vi "decoupled_gains_vec.vi"(11 "Gain":T1 {"Rz" min=0 max=1 step=0.1 format="%#_3p"; "Rxy" min=0 max=1 step=0.1 format="%#_3p"; "Z" min=0 max=1 step=0.1 format="%#_3p"; "XY" min=0 max=1 step=0.1 format="%#_3p"}) -> (3 "Decoupled":sgl[](array[numeric]) format="%#_3g")   [LabVIEW 2013]
uses:
  decoupled_gain.ctl
panel:
  # "Convert cluster representation of controller mode gains into flat vector."
  # "----------XY----------"
  # "----------RxRy----------"
  # "Z"
  # "Rz"
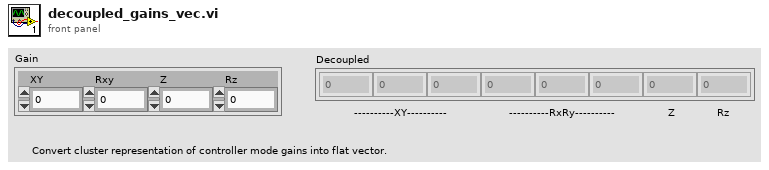
[diagram p1: front panel]
types:
  T1 = typedef "decoupled_gain.ctl" = cluster{"XY":sgl, "Rxy":sgl, "Z":sgl, "Rz":sgl}
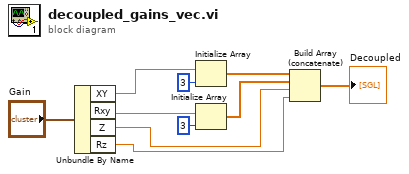
[diagram p0: block diagram]
diagram:
  n1 = Unbundle By Name("Gain") -> ("XY"=w2:sgl, "Rxy"=w5:sgl, "Z"=w8:sgl, "Rz"=w9:sgl)
  n2 = Initialize Array(w2, 3 ("dimension size")) -> (w6:sgl[])
  n3 = Initialize Array(w5, 3 ("dimension size")) -> (w7:sgl[])
  n4 = Build Array (concatenate)(w6, w7, w8, w9) -> (→"Decoupled":sgl[])
